vi "Autotest_Instr.vi"(8 "error in (no error)":errorcluster caption="entrée d'erreur (pas d'erreur)", 11 "Class DIO en entrée":refnum<class "Class Instrument Log_File.lvclass">) -> (0 "error out":errorcluster caption="sortie d'erreur", 3 "Class DIO en Sortie":refnum<class "Class Instrument Log_File.lvclass">)   [LabVIEW 2020, in "Library Instrument & Equipement.lvlib" / "Library Instruments.lvlib" / "Class Instrument Log_File.lvclass"]
uses:
  Class Instrument Log_File.lvclass
  C:/Users/ngarcin/OneDrive - Altyor/Standard TB/Class/Instrument/Instrument (Default)/Class Instrument (Default).lvclass
  Instrument (Default)/Class Instrument (Default).lvclass
  Class Instrument Log_File.lvclass/Class Instrument Log_File.ctl
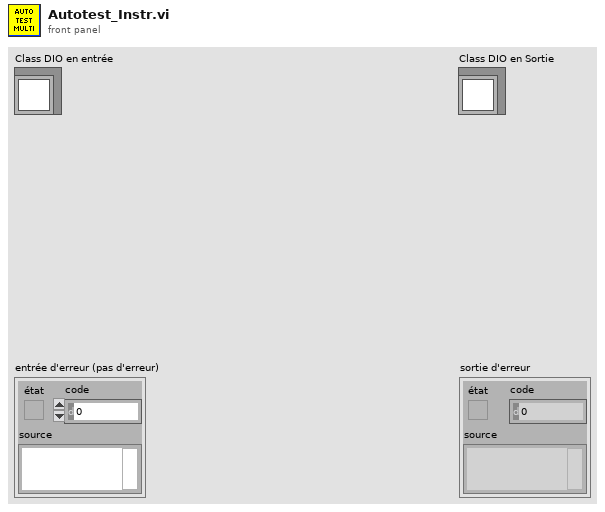
[diagram p1: front panel]
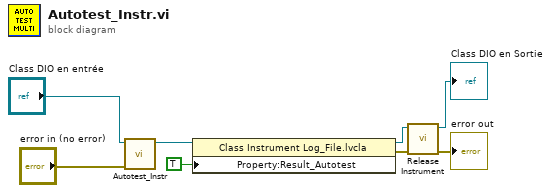
[diagram p0: block diagram]
diagram:
  n1 = call-parent "Autotest_Instr.vi"("error in (no error)"="error in (no error)", "Class Instrument (Default) en entrée"="Class DIO en entrée") -> ("Class Instrument (Default) en sortie"=w2:refnum<class "Class Instrument Log_File.lvclass">)  [unwired: 8 in, 1 out]
  n2 = property class="Class Instrument Log_File.lvcla"(reference=w2, "Property:Result_Autotest"=TRUE ("Result_Autotest")) -> (reference out=w4:refnum<class "Class Instrument Log_File.lvclass">, error out=w6:errorcluster)  [unwired: 1 in]
  n3 = call-dynamic "Release Instrument.vi"("error in (no error)"=w6, "Class Instrument (Default) en entrée"=w4) -> ("error out"=→"error out":errorcluster, "Class Instrument (Default) en sortie"=→"Class DIO en Sortie":refnum<class "Class Instrument Log_File.lvclass">)  [unwired: 8 in]
